vi "Punto 2.vi"() -> ()   [LabVIEW 2020]
panel:
  in  "Stop buttom":bool
  in  "Temperature":dbl
  out "New temperature":dbl
  in  "Operate":bool
  in  "Scale of temperature #2":string(combo)
  in  "Scale of temperature #1":string(combo)
  # "This program was created by Juan Bermúdez from the Army Aviation School\nat the Aircraft Engineering of the assignature of Programation II"
  # "How to use the software?:\n1- First, select the scale of temperature original.\n2- Second, select the new scale of temperature.\n3- Third, write the value of the temperature.\n4- Forth, push the buttom called = ''Operate''.\n5- Fifth, if you want to stop the software, push the buttom called = ''Stop buttom''.\n Enjoy the software :)"
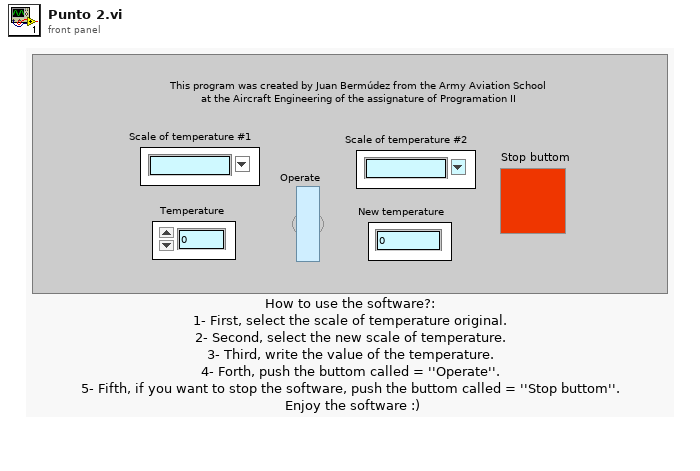
[diagram p1: front panel]
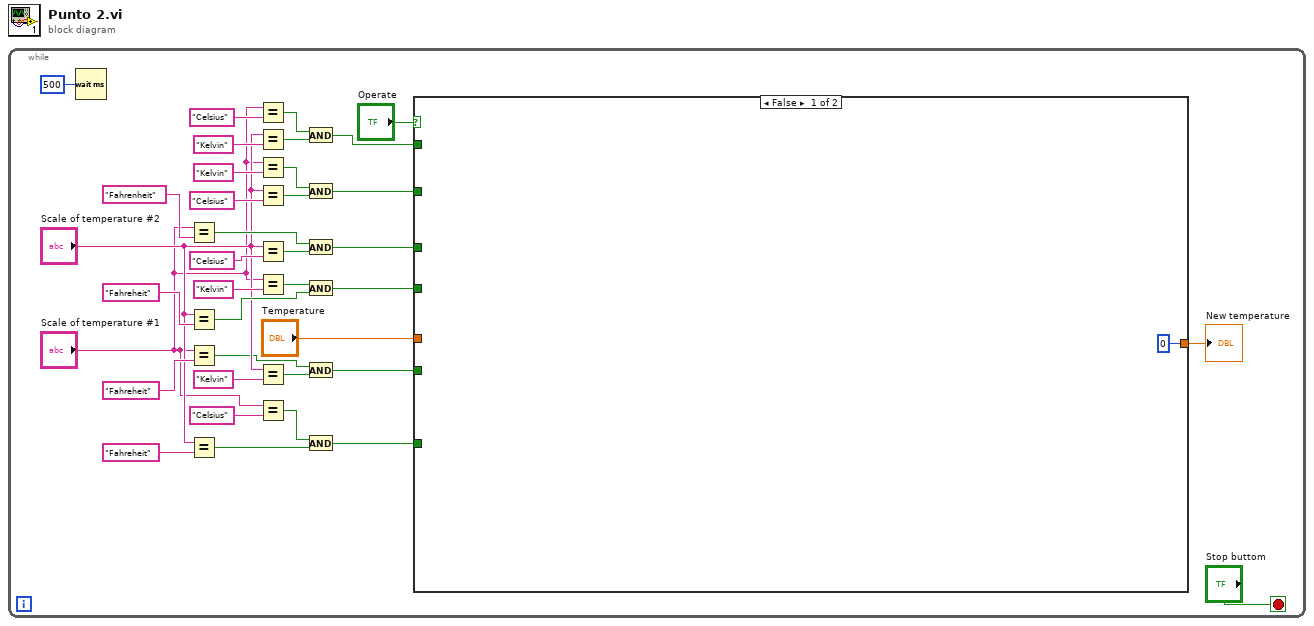
[diagram p0: block diagram]
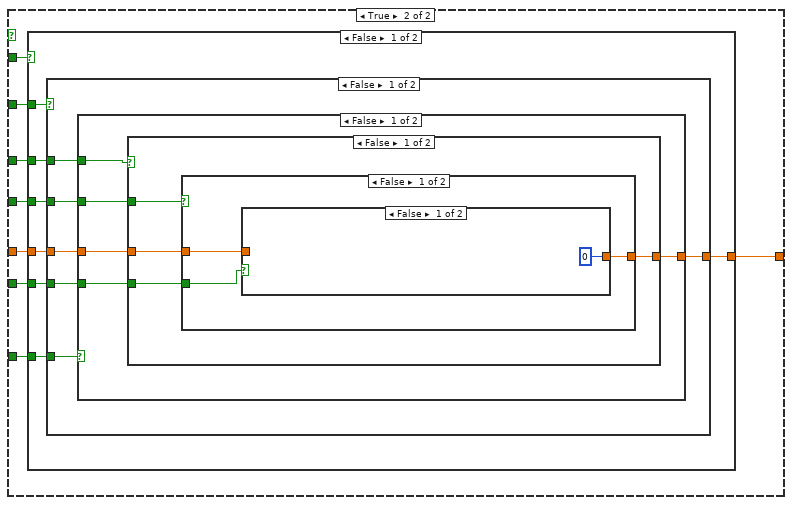
[diagram p2: hidden frame]
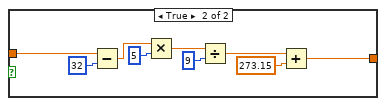
[diagram p3: hidden frame]
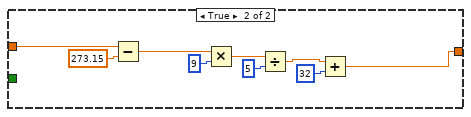
[diagram p4: hidden frame]
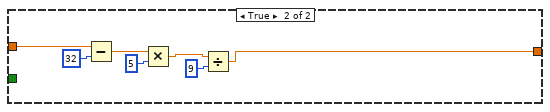
[diagram p5: hidden frame]
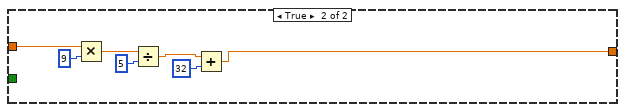
[diagram p6: hidden frame]
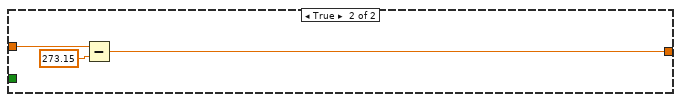
[diagram p7: hidden frame]
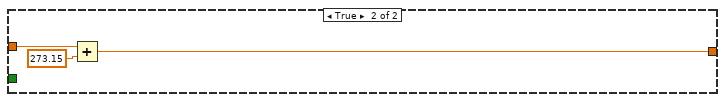
[diagram p8: hidden frame]
diagram:
  n1 = while {
    stop <- "Stop buttom" stop-if-true
    n2 = Wait (ms)(milliseconds to wait=500) -> ()  [unwired: 1 out]
    n3 = Equal?(x="Scale of temperature #1", y="Fahrenheit") -> (x = y?=w17:bool)
    n4 = Equal?(x="Scale of temperature #2", y="Fahreheit") -> (x = y?=w10:bool)
    n5 = Equal?(x="Scale of temperature #1", y="Fahreheit") -> (x = y?=w5:bool)
    n6 = Equal?(x="Scale of temperature #2", y="Fahreheit") -> (x = y?=w20:bool)
    n7 = Equal?(x="Scale of temperature #1", y="Celsius") -> (x = y?=w32:bool)
    n8 = Equal?(x="Scale of temperature #2", y="Kelvin") -> (x = y?=w31:bool)
    n9 = Equal?(x="Scale of temperature #1", y="Kelvin") -> (x = y?=w28:bool)
    n10 = Equal?(x="Scale of temperature #2", y="Celsius") -> (x = y?=w25:bool)
    n11 = Equal?(x="Scale of temperature #2", y="Celsius") -> (x = y?=w15:bool)
    n12 = Equal?(x="Scale of temperature #1", y="Kelvin") -> (x = y?=w11:bool)
    n13 = Equal?(x="Scale of temperature #2", y="Kelvin") -> (x = y?=w4:bool)
    n14 = Equal?(x="Scale of temperature #1", y="Celsius") -> (x = y?=w21:bool)
    n15 = And(x=w32, y=w31) -> (x .and. y?=w30:bool)
    n16 = And(x=w28, y=w25) -> (x .and. y?=w24:bool)
    n17 = And(x=w17, y=w15) -> (x .and. y?=w14:bool)
    n18 = And(x=w11, y=w10) -> (x .and. y?=w9:bool)
    n19 = And(x=w5, y=w4) -> (x .and. y?=w3:bool)
    n20 = And(x=w21, y=w20) -> (x .and. y?=w19:bool)
    n21 = case shown="False" "Operate" {
      tunnel: [0 w44] -> w34
      tunnel: w30 -> [_ w46]
      tunnel: "Temperature" -> [_ w45]
      tunnel: w24 -> [_ w43]
      tunnel: w19 -> [_ w42]
      tunnel: w14 -> [_ w41]
      tunnel: w9 -> [_ w40]
      tunnel: w3 -> [_ w39]
      frame False {
      }
      frame True {
        n22 = case shown="False" w46 {
          tunnel: w45 -> [w52 w110]
          tunnel: [w51 w108] -> w44
          tunnel: w43 -> [w53 _]
          tunnel: w42 -> [w50 _]
          tunnel: w41 -> [w49 _]
          tunnel: w40 -> [w48 _]
          tunnel: w39 -> [w47 _]
          frame False {
            n23 = case shown="False" w53 {
              tunnel: w52 -> [w58 w107]
              tunnel: [w57 w105] -> w51
              tunnel: w50 -> [w59 _]
              tunnel: w49 -> [w56 _]
              tunnel: w48 -> [w55 _]
              tunnel: w47 -> [w54 _]
              frame False {
                n24 = case shown="False" w59 {
                  tunnel: w58 -> [w63 w104]
                  tunnel: [w62 w98] -> w57
                  tunnel: w56 -> [w64 _]
                  tunnel: w55 -> [w61 _]
                  tunnel: w54 -> [w60 _]
                  frame False {
                    n25 = case shown="False" w64 {
                      tunnel: w63 -> [w67 w97]
                      tunnel: [w66 w91] -> w62
                      tunnel: w61 -> [w68 _]
                      tunnel: w60 -> [w65 _]
                      frame False {
                        n26 = case shown="False" w68 {
                          tunnel: w67 -> [w70 w90]
                          tunnel: [w69 w82] -> w66
                          tunnel: w65 -> [w71 _]
                          frame False {
                            n27 = case shown="False" w71 {
                              tunnel: w70 -> [_ w81]
                              tunnel: [0 w73] -> w69
                              frame False {
                              }
                              frame True {
                                n28 = Subtract(x=w81, y=32) -> (x-y=w79:dbl)
                                n29 = Multiply(x=w79, y=5) -> (x*y=w77:dbl)
                                n30 = Divide(x=w77, y=9) -> (x/y=w75:dbl)
                                n31 = Add(x=w75, y=273.15) -> (x+y=w73:dbl)
                              }
                            }
                          }
                          frame True {
                            n32 = Subtract(x=w90, y=273.15) -> (x-y=w88:dbl)
                            n33 = Multiply(x=w88, y=9) -> (x*y=w86:dbl)
                            n34 = Divide(x=w86, y=5) -> (x/y=w84:dbl)
                            n35 = Add(x=w84, y=32) -> (x+y=w82:dbl)
                          }
                        }
                      }
                      frame True {
                        n36 = Subtract(x=w97, y=32) -> (x-y=w95:dbl)
                        n37 = Multiply(x=w95, y=5) -> (x*y=w93:dbl)
                        n38 = Divide(x=w93, y=9) -> (x/y=w91:dbl)
                      }
                    }
                  }
                  frame True {
                    n39 = Multiply(x=w104, y=9) -> (x*y=w102:dbl)
                    n40 = Divide(x=w102, y=5) -> (x/y=w100:dbl)
                    n41 = Add(x=w100, y=32) -> (x+y=w98:dbl)
                  }
                }
              }
              frame True {
                n42 = Subtract(x=w107, y=273.15) -> (x-y=w105:dbl)
              }
            }
          }
          frame True {
            n43 = Add(x=w110, y=273.15) -> (x+y=w108:dbl)
          }
        }
      }
    }
    "New temperature" <- w34
  }
